vi "FileIO_CreateTextFile.vi"(0 "Target Folder Path":path, 5 "File Name (add .txt)":string, 7 "Text String":string, 11 "Error In":errorcluster) -> (4 "File Path":path, 15 "Error Out":errorcluster)   [LabVIEW 2016]
doc: "Creates a text file with desired file name to desired folder, and writes text to this file. Text to be written to the file is reccomended but not required.\n\nNote: It only will create a new file(not replace existing or open existing etc). If file alreday exists in directory it will error."
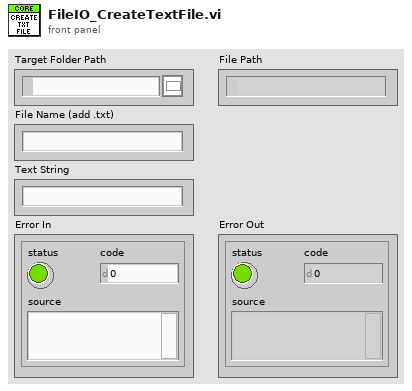
[diagram p1: front panel]
types:
  T1 = enum16{"open", "replace", "create", "open or create", "replace or create", "replace or create with confirmation"}
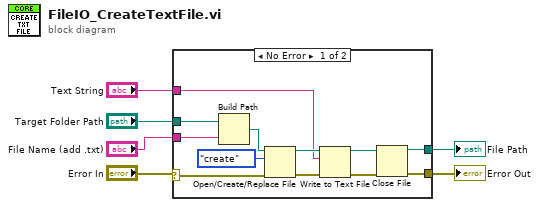
[diagram p0: block diagram]
diagram:
  n1 = case shown="No Error" "Error In" {
    selector: "Error In" -> [w8 w19]
    tunnel: [w16 w19] -> w6
    tunnel: "Target Folder Path" -> [w15 _]
    tunnel: "File Name (add .txt)" -> [w14 _]
    tunnel: "Text String" -> [w11 _]
    tunnel: [w9 _] -> w2
    frame No Error {
      n2 = Build Path(base path=w15, name or relative path=w14) -> (appended path=w13:path)
      n3 = Open/Create/Replace File(file path (use dialog)=w13, error in=w8, operation (0:open)=T1."create") -> (refnum out=w12:refnum<file>, error out=w18:errorcluster)  [unwired: 3 in, 1 out]
      n4 = Write to Text File(file (use dialog)=w12, text=w11, error in=w18) -> (refnum out=w10:refnum<file>, error out=w17:errorcluster)  [unwired: 1 in, 1 out]
      n5 = Close File(refnum=w10, error in=w17) -> (path=w9:path, error out=w16:errorcluster)
    }
    frame Error {
    }
  }
  "Error Out" <- w6
  "File Path" <- w2
